vi "Create Date Time String.vi"(8 "Error In":errorcluster) -> (0 "Error Out":errorcluster, 2 "Date/Time String":string)   [LabVIEW 2014]
doc: "Creates a string containing the current date and time (i.e. Apr-21-2012 Time 11 38 PM)."
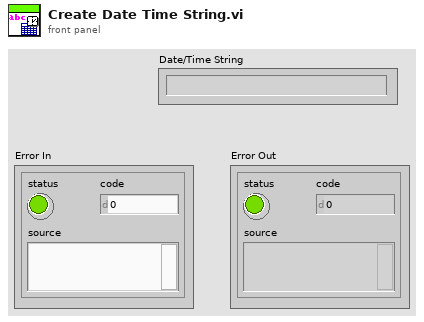
[diagram p1: front panel]
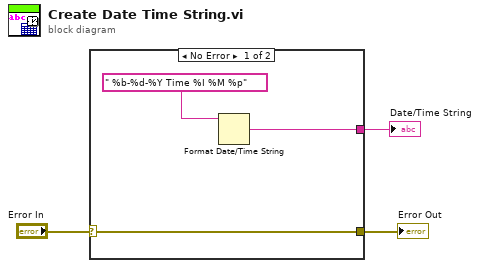
[diagram p0: block diagram]
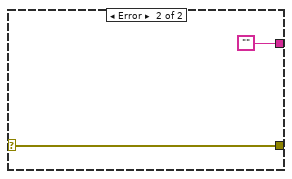
[diagram p2: hidden frame]
diagram:
  n1 = case shown="No Error" "Error In" {
    selector: "Error In" -> [w5 w7]
    tunnel: [w5 w7] -> w2
    tunnel: [w4 ""] -> w1
    frame No Error {
      n2 = Format Date/Time String(time format string (%c)=" %b-%d-%Y Time %I %M %p") -> (date/time string=w4:string)  [unwired: 2 in]
    }
    frame Error {
    }
  }
  "Error Out" <- w2
  "Date/Time String" <- w1
